vi "FGV Komm Status.vi"(6 "Aktionen":T1, 11 "lebt PC?":bool) -> (3 "lebt PC?":bool)   [LabVIEW 2020, in "Kommunikation mit PC.lvlib"]
uses:
  Kommunikation mit PC.lvlib
  FGV Komm Status Aktionen.ctl
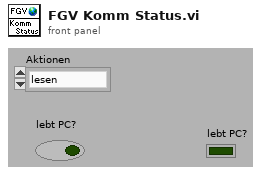
[diagram p1: front panel]
types:
  T1 = typedef "Kommunikation mit PC.lvlib/FGV Komm Status Aktionen.ctl" = enum16{"lesen", "lebt PC?"}
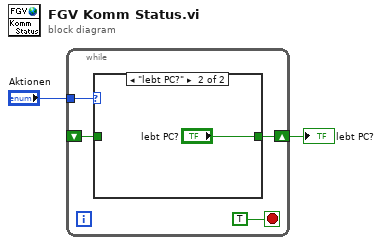
[diagram p0: block diagram]
diagram:
  n1 = while {
    tunnel: "Aktionen" -> [w5]
    shift-right: [w4] -> w1
    shift-left: _ -> [w3]
    stop <- TRUE stop-if-true
    n2 = case shown="\"lebt PC?\"" w5 {
      tunnel: [w7 "lebt PC?"] -> w4
      tunnel: w3 -> [w7 _]
      frame "lesen", Default {
      }
      frame "lebt PC?" {
      }
    }
  }
  "lebt PC?" <- w1
